vi "Publish.vi"(8 "error in (no error)":errorcluster, 10 "PUBLISH":refnum<class "PUBLISH.lvclass">, 11 "Subscription in":refnum<class "Subscription.lvclass">) -> (0 "error out":errorcluster, 3 "Subscription out":refnum<class "Subscription.lvclass">)   [LabVIEW 2013, in "MQTT Base.lvlib" / "Subscription.lvclass"]
uses:
  Subscription.lvclass
  <vilib>/LabVIEW Open Source Project/MQTT Control Packets/Control Packets/PUBLISH/PUBLISH.lvclass
  Base Class/Response -- cluster.ctl
  <vilib>/LabVIEW Open Source Project/MQTT Control Packets/Control Packets/ControlPacket/ControlPacket.lvclass
  Subscription.lvclass/Subscription.ctl
  TopicFilter/TopicFilter.lvclass
  Base Class/MQTT_Base.lvclass
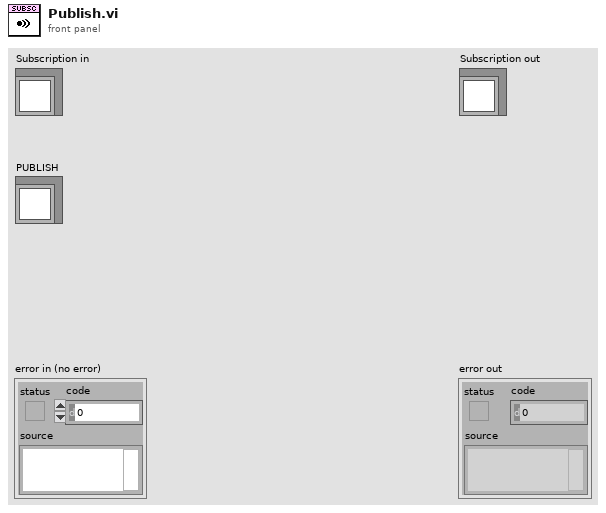
[diagram p1: front panel]
types:
  T1 = typedef "MQTT Base.lvlib/MQTT_Base.lvclass/Response -- cluster.ctl" = cluster{"Packet":refnum<class "ControlPacket.lvclass">, "Protocol Error":errorcluster, "disconnect session":bool, "[ACK]":refnum<notifier>[]}
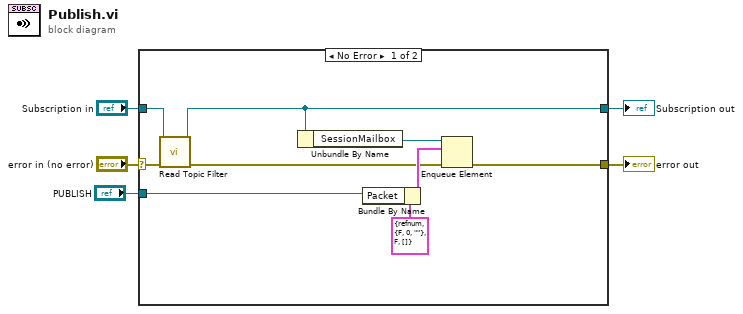
[diagram p0: block diagram]
diagram:
  n1 = case shown="No Error" "error in (no error)" {
    selector: "error in (no error)" -> [w9 w16]
    tunnel: [w10 w16] -> w4
    tunnel: [w6 w15] -> w2
    tunnel: "Subscription in" -> [w7 w15]
    tunnel: "PUBLISH" -> [w12 _]
    frame No Error {
      n2 = call "Read Topic Filter.vi"("error in (no error)"=w9, "Subscription in"=w7) -> ("error out"=w8:errorcluster, "Subscription out"=w6:refnum<class "Subscription.lvclass">)  [unwired: 6 in, 2 out]
      n3 = Unbundle By Name(w6) -> ("SessionMailbox"=w14:refnum<queue>)
      n4 = Bundle By Name(cluster=T1 {"Packet"=refnum, "Protocol Error"={"status"=FALSE, "code"=0, "source"=""}, "disconnect session"=FALSE, "[ACK]"=[]} ("element"), "Packet"=w12) -> (w11:T1)
      n5 = Enqueue Element(queue=w14, element=w11, error in (no error)=w8) -> (error out=w10:errorcluster)  [unwired: 1 in, 2 out]
    }
    frame Error {
    }
  }
  "error out" <- w4
  "Subscription out" <- w2
